vi "stoperaseAO_img.vi"   [LabVIEW 2015]
uses:
  waveforms/usedAOindepofwf.vi
  Misc/add channel to active arrayv2.vi
  Objects/2pparameters.vi
types:
  T1 = cluster{"AO":refnum<k21>[], "E_AO":errorcluster[]}
  T2 = typedef "XYZStage.lvlib/XYZStage Configuration.ctl" = cluster{"VISA resource name":refnum<visa-resource-name>, "Timeout (3sec)":u32}
  T3 = cluster{"StageS":i32, "StageL":i32, "currmeas data dir":path, "image OD":u16, "contour OD":u16, "point OD":u16, "AOlines":tag[], "AIlines":tag[], "CI lines":tag[], "DO lines":tag[], "AO names":string[], "CI names":string[], "AI names":string[], "DO names":string[], "CIextensions":string[], "AIextensions":string[], "Voltage to Ygalvo":i32, "Voltage to Xgalvo":i32, "Voltage to patch":i32, "640 shutter":i32, "2P shutter":i32, "LT timestamp":u32, "Vp":i32, "Ip":i32, "camera trigger":i32, "master data dir":path, "voltage to Zpos":i32, "Vto2P":i32, "640 AO":i32, "488 AO":i32, "532 AO":i32, "640TTL":u32, "488TTL":u32, "532TTL":u32, "Device 1 sampleclock out":tag, "Device 1 Starttrigger out":tag, "Device 2 sampleclock in":tag, "Device 2 StartTrigger in ":tag, "2PODTTL":u32, "488 shutter":u32, "LCVR red":u32, "LCVR blue":u32, "Sutter Stage Config":T2, "Device 1 ext sampleclock in (100Khz)":tag}
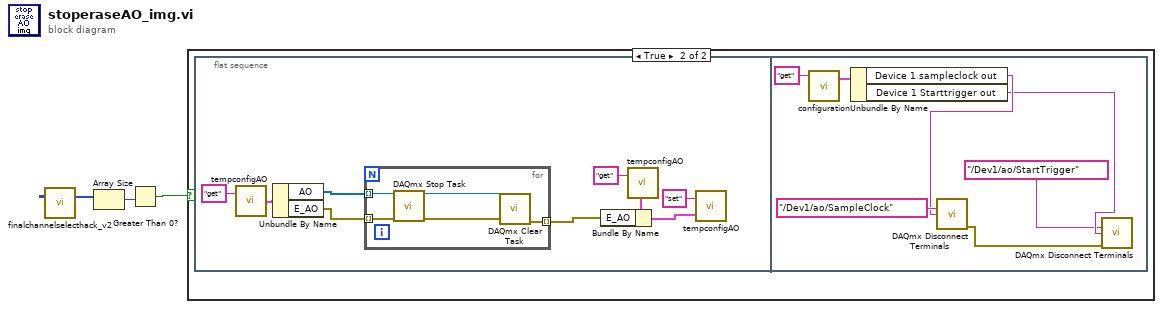
[diagram p0: block diagram]
diagram:
  n1 = call "finalchannelselecthack_v2.vi"() -> ("devices"=w1:u32[])  [unwired: 1 in, 1 out]
  n2 = Array Size(array=w1) -> (size(s)=w3:i32)
  n3 = Greater Than 0?(x=w3) -> (x > 0?=w2:bool)
  n4 = case shown="True" w2 {
    frame False {
    }
    frame True {
      n5 = flat-sequence {
        frame #0 {
          n6 = call "tempconfigAO.vi"("command"="get") -> ("Temp Config out"=w11:T1)  [unwired: 1 in]
          n7 = Unbundle By Name(w11) -> ("AO"=w5:refnum<k21>[], "E_AO"=w4:errorcluster[])
          n8 = for {
            tunnel: [w17] -> w7 mode=indexing
            tunnel: w5 -> [w16] mode=indexing
            tunnel: w4 -> [w13] mode=indexing
            n9 = call <vilib>:"DAQmx Stop Task.vi"("task/channels in"=w16, "error in"=w13) -> ("task out"=w15:refnum<k21>, "error out"=w14:errorcluster)  [unwired: 12 in]
            n10 = call <vilib>:"DAQmx Clear Task.vi"("task in"=w15, "error in"=w14) -> ("error out"=w17:errorcluster)  [unwired: 13 in]
          }
          n11 = call "tempconfigAO.vi"("command"="get") -> ("Temp Config out"=w8:T1)  [unwired: 1 in]
          n12 = Bundle By Name(cluster=w8, "E_AO"=w7) -> (w6:T1)
          n13 = call "tempconfigAO.vi"("Temp Config in"=w6, "command"="set") -> ()  [unwired: 1 out]
        }
        frame #1 {
          n14 = call "configuration.vi"("command"="get") -> ("config out"=w24:T3)  [unwired: 2 in, 1 out]
          n15 = Unbundle By Name(w24) -> ("Device 1 sampleclock out"=w21:tag, "Device 1 Starttrigger out"=w20:tag)
          n16 = call <vilib>:"DAQmx Disconnect Terminals.vi"("source terminal"=tag "/Dev1/ao/SampleClock", "destination terminal"=w21) -> ("error out"=w18:errorcluster)  [unwired: 13 in]
          n17 = call <vilib>:"DAQmx Disconnect Terminals.vi"("source terminal"=tag "/Dev1/ao/StartTrigger", "destination terminal"=w20, "error in"=w18) -> ()  [unwired: 12 in, 1 out]
        }
      }
    }
  }
